vi "Format Path and Filename.vi"(8 "error in":errorcluster, 11 "Data in":refnum<class "Data.lvclass">) -> (0 "error out":errorcluster, 3 "Data out":refnum<class "Data.lvclass">)   [LabVIEW 2019, in "Data.lvclass"]
uses:
  Data.lvclass
  Typedefs/Operation--enum.ctl
panel:
  out "path in":path
  out "formatted path":path
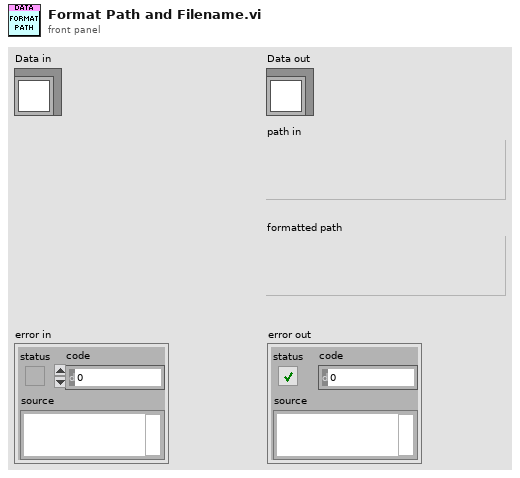
[diagram p1: front panel]
types:
  T1 = typedef "Data.lvclass/Operation--enum.ctl" = enum16{"Read", "Write", "Write + Append"}
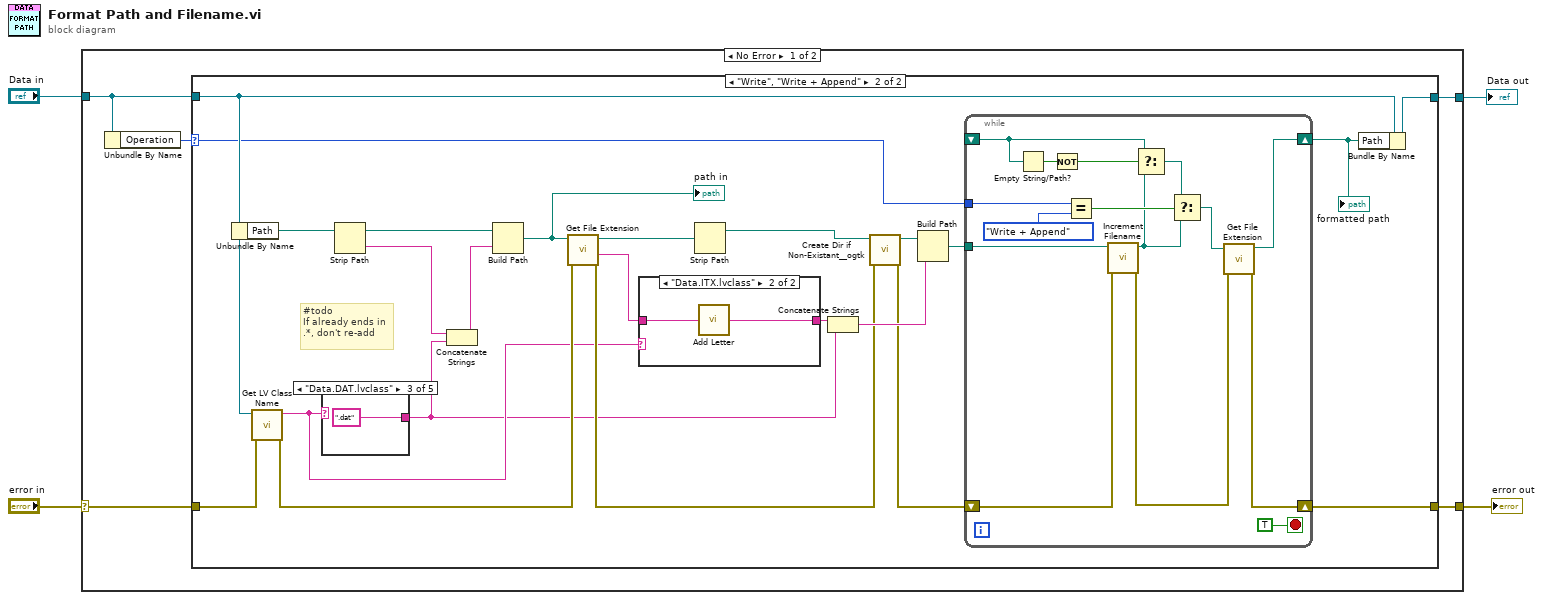
[diagram p0: block diagram]
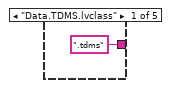
[diagram p4: hidden frame]
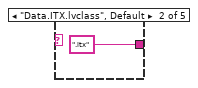
[diagram p5: hidden frame]
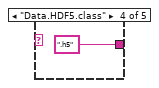
[diagram p6: hidden frame]
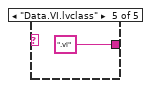
[diagram p7: hidden frame]
diagram:
  n1 = case shown="No Error" "error in" {
    selector: "error in" -> [w8 w59]
    tunnel: [w9 w59] -> w4
    tunnel: "Data in" -> [w6 w58]
    tunnel: [w7 w58] -> w1
    frame No Error {
      n2 = Unbundle By Name(w6) -> ("Operation"=w5:T1)
      n3 = case shown="\"Write\", \"Write + Append\"" w5 {
        selector: w5 -> [_ w19]
        tunnel: [w10 w32] -> w9
        tunnel: w8 -> [w10 w24]
        tunnel: [w11 w22] -> w7
        tunnel: w6 -> [w11 w21]
        frame "Read", Default {
        }
        frame "Write", "Write + Append" {
          # "#todo\nIf already ends in\n.*, don't re-add"
          n4 = Unbundle By Name(w21) -> ("Path"=w18:path)
          n5 = call <vilib>:"Get LV Class Name.vi"("error in (no error)"=w24, "object"=w21) -> ("error out"=w23:errorcluster, "class name"=w14:string)  [unwired: 8 in]
          n6 = case shown="\"Data.DAT.lvclass\"" w14 {
            tunnel: [".tdms" ("string") ".itx" ("string") ".dat" ("string") ".h5" ("string") ".vi" ("string")] -> w13
            frame "Data.TDMS.lvclass" {
            }
            frame "Data.ITX.lvclass", Default {
            }
            frame "Data.DAT.lvclass" {
            }
            frame "Data.HDF5.class" {
            }
            frame "Data.VI.lvclass" {
            }
          }
          n7 = Strip Path(path=w18) -> (stripped path=w17:path, name=w12:string)
          n8 = Concatenate Strings(w12, w13) -> (w15:string)
          n9 = Build Path(base path=w17, name or relative path=w15) -> (appended path=w16:path)
          "path in" <- w16
          n10 = call <vilib>:"Get File Extension.vi"("error in (no error)"=w23, "file"=w16) -> ("error out"=w26:errorcluster, "filename without extension"=w27:string, "dup file"=w29:path)  [unwired: 7 out]
          n11 = case shown="\"Data.ITX.lvclass\"" w14 {
            tunnel: [w35 w37] -> w33
            tunnel: w27 -> [w35 w36]
            frame Default {
            }
            frame "Data.ITX.lvclass" {
              n12 = call "Add Letter.vi"("string"=w36) -> ("result string"=w37:string)
            }
          }
          n13 = Strip Path(path=w29) -> (stripped path=w28:path)  [unwired: 1 out]
          n14 = Concatenate Strings(w33, w13) -> (w34:string)
          n15 = call "Create Dir if Non-Existant__ogtk.vi"("error in (no error)"=w26, "Directory Path"=w28) -> ("error out"=w31:errorcluster, "dup Directory Path"=w25:path)  [unwired: 7 in, 1 out]
          n16 = Build Path(base path=w25, name or relative path=w34) -> (appended path=w30:path)
          n17 = while {
            tunnel: w19 -> [w42]
            tunnel: w30 -> [w40]
            shift-right: [w46] -> w20
            shift-left: _ -> [w49]
            shift-right: [w48] -> w32
            shift-left: w31 -> [w45]
            stop <- TRUE stop-if-true
            n18 = Empty String/Path?(string/path=w49) -> (empty?=w51:bool)
            n19 = Not(x=w51) -> (.not. x?=w50:bool)
            n20 = Equal?(x=w42, y=Operation--enum."Write + Append" ("Operation")) -> (x = y?=w41:bool)
            n21 = call "Increment Filename.vi"("error in (no error)"=w45, "Path"=w40) -> ("error out"=w44:errorcluster, "Modified Path"=w39:path)  [unwired: 8 in]
            n22 = Select(t=w49, s=w50, f=w39) -> (s? t:f=w38:path)
            n23 = Select(t=w38, s=w41, f=w39) -> (s? t:f=w47:path)
            n24 = call <vilib>:"Get File Extension.vi"("error in (no error)"=w44, "file"=w47) -> ("error out"=w48:errorcluster, "dup file"=w46:path)  [unwired: 8 out]
          }
          "formatted path" <- w20
          n25 = Bundle By Name(cluster=w21, "Path"=w20) -> (w22:refnum<class "Data.lvclass">)
        }
      }
    }
    frame Error {
    }
  }
  "error out" <- w4
  "Data out" <- w1
